vi "cXB_trt-0-init.vi"(11 "cX-e":T1) -> (3 "cX-s":T1)   [LabVIEW 2010]
uses:
  lv_04/commandes/cX.ctl
  lv_04/commandes/cSTA_varid.ctl
  lv_04/commandes/c_TDMS_ch_variable.ctl
  lv_04/commandes/c_TDMS_ch_donnees.ctl
  lv_04/commandes/c0-var-n.ctl
  lv_04/commandes/cSTA_num_do_cr.ctl
  lv_04/commandes/c02-do-num.ctl
  lv_04/commandes/c04-stat-num.ctl
  lv_04/commandes/cSTA_txt_do_cr.ctl
  lv_04/commandes/c02-do-txt.ctl
  lv_04/commandes/c04-stat-txt.ctl
  lv_04/commandes/cSTA_dist.ctl
  lv_04/commandes/c03-dist-S.ctl
  lv_04/commandes/c0-dist-xy.ctl
  lv_04/commandes/c03-dist-T.ctl
  lv_04/commandes/c03-dist-SPC.ctl
  lv_02/lv_02.lvlib
  lv_04/lv_04.lvlib
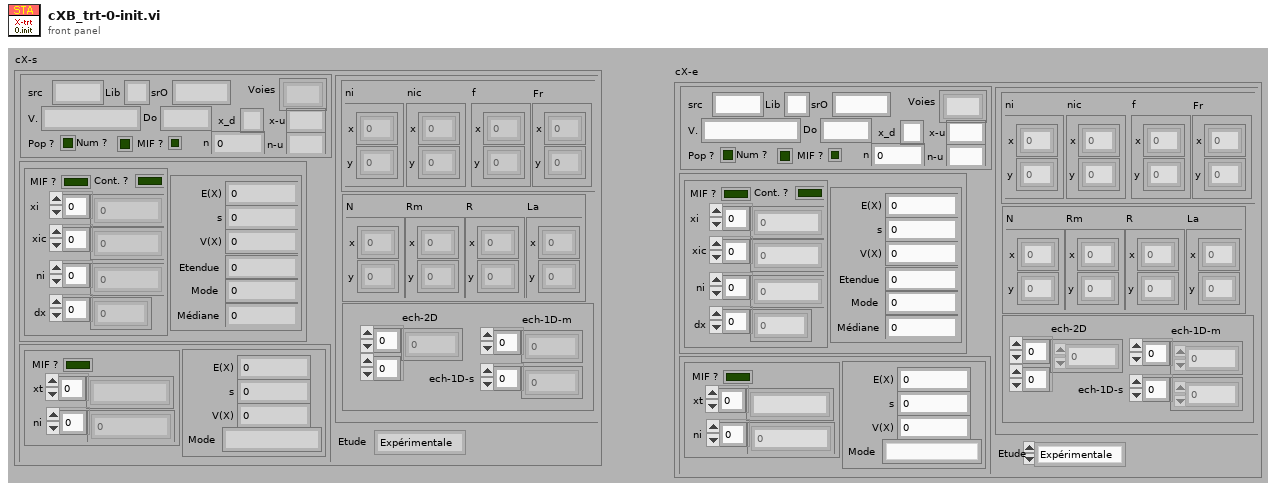
[diagram p1: front panel]
types:
  T1 = typedef "lv_04.lvlib/cX.ctl" = cluster{"src":T2, "num":T6, "txt":T9, "dist":T12, "Etude":enum16{"Expérimentale", "Modèle"}}
  T2 = typedef "lv_04.lvlib/cSTA_varid.ctl" = cluster{"src":string, "Lib":string, "srO":string, "V.":T3, "Voies":string[], "Do":T4, "n":T5, "Num ?":bool, "Pop ?":bool, "x_d":string, "x-u":string, "n-u":string, "MIF ?":bool}
  T3 = typedef "lv_04.lvlib/c_TDMS_ch_variable.ctl" = string
  T4 = typedef "lv_04.lvlib/c_TDMS_ch_donnees.ctl" = string
  T5 = typedef "lv_04.lvlib/c0-var-n.ctl" = i32
  T6 = typedef "lv_04.lvlib/cSTA_num_do_cr.ctl" = cluster{"do":T7, "sta":T8}
  T7 = typedef "lv_04.lvlib/c02-do-num.ctl" = cluster{"MIF ?":bool, "Cont. ?":bool, "xi":dbl[], "xic":dbl[], "ni":u32[], "dx":dbl[]}
  T8 = typedef "lv_04.lvlib/c04-stat-num.ctl" = cluster{"E(X)":dbl, "s":dbl, "V(X) ":dbl, "Etendue":dbl, "Mode":dbl, "Médiane":dbl}
  T9 = typedef "lv_04.lvlib/cSTA_txt_do_cr.ctl" = cluster{"do":T10, "sta":T11}
  T10 = typedef "lv_04.lvlib/c02-do-txt.ctl" = cluster{"xt":string[], "ni":dbl[], "MIF ?":bool}
  T11 = typedef "lv_04.lvlib/c04-stat-txt.ctl" = cluster{"E(X)":dbl, "s":dbl, "V(X) ":dbl, "Mode":string}
  T12 = typedef "lv_04.lvlib/cSTA_dist.ctl" = cluster{"S":T13, "T":T15, "spc":T16}
  T13 = typedef "lv_04.lvlib/c03-dist-S.ctl" = cluster{"nic":T14, "f":T14, "Fr":T14, "ni":T14}
  T14 = typedef "lv_04.lvlib/c0-dist-xy.ctl" = cluster{"x":dbl[], "y":dbl[]}
  T15 = typedef "lv_04.lvlib/c03-dist-T.ctl" = cluster{"N":T14, "Rm":T14, "R":T14, "La":T14}
  T16 = typedef "lv_04.lvlib/c03-dist-SPC.ctl" = cluster{"ech-2D":dbl[][], "ech-1D-m":dbl[], "ech-1D-s":dbl[]}
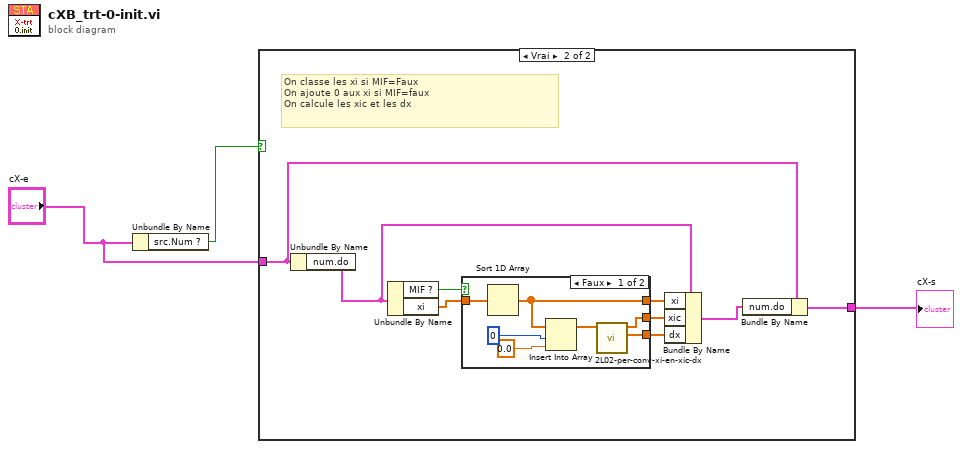
[diagram p0: block diagram]
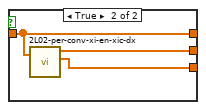
[diagram p3: hidden frame]
diagram:
  n1 = Unbundle By Name("cX-e") -> ("src.Num ?"=w3:bool)
  n2 = case shown="Vrai" w3 {
    tunnel: "cX-e" -> [w4 w7]
    tunnel: [w4 w5] -> w2
    frame False {
    }
    frame True {
      # "On classe les xi si MIF=Faux\nOn ajoute 0 aux xi si MIF=faux\nOn calcule les xic et les dx"
      n3 = Unbundle By Name(w7) -> ("num.do"=w8:T7)
      n4 = Unbundle By Name(w8) -> ("MIF ?"=w13:bool, "xi"=w9:dbl[])
      n5 = case shown="Faux" w13 {
        tunnel: w9 -> [w20 w21]
        tunnel: [w19 w21] -> w10
        tunnel: [w15 w23] -> w11
        tunnel: [w14 w22] -> w12
        frame False {
          n6 = Sort 1D Array(array=w20) -> (sorted array=w19:dbl[])
          n7 = Insert Into Array(array=w19, index=0 ("indice"), new element=0.0 ("nouvel élément/sous-tableau")) -> (w16:dbl[])
          n8 = call "2L02-per-conv-xi-en-xic-dx.vi"("xi"=w16) -> ("dx"=w14:dbl[], "xic"=w15:dbl[])  [unwired: 7 in]
        }
        frame True {
          n9 = call "2L02-per-conv-xi-en-xic-dx.vi"("xi"=w21) -> ("dx"=w22:dbl[], "xic"=w23:dbl[])  [unwired: 7 in]
        }
      }
      n10 = Bundle By Name(cluster=w8, "xi"=w10, "xic"=w11, "dx"=w12) -> (w6:T7)
      n11 = Bundle By Name(cluster=w7, "num.do"=w6) -> (w5:T1)
    }
  }
  "cX-s" <- w2
